vi "setUnderlineToDocument.vi"(8 "error in (no error)":errorcluster, 11 "xwpfRun in":refnum<class "xwpfRun.lvclass">) -> (0 "error out":errorcluster, 3 "xwpfRun out":refnum<class "xwpfRun.lvclass">)   [LabVIEW 2017, in "Word_Specific.lvlib" / "xwpfRun.lvclass"]
uses:
  xwpfRun.lvclass
  xwpfRun.lvclass/xwpfRun.ctl
  C:/Users/Neo/Desktop/Dev_Tools_BR/LabVIEW_NPOI/lib/NPOI 2.1.1/NPOI.OOXML.dll
  lib/NPOI 2.1.1/NPOI.OOXML.dll
  Styles/Style/Style.lvclass
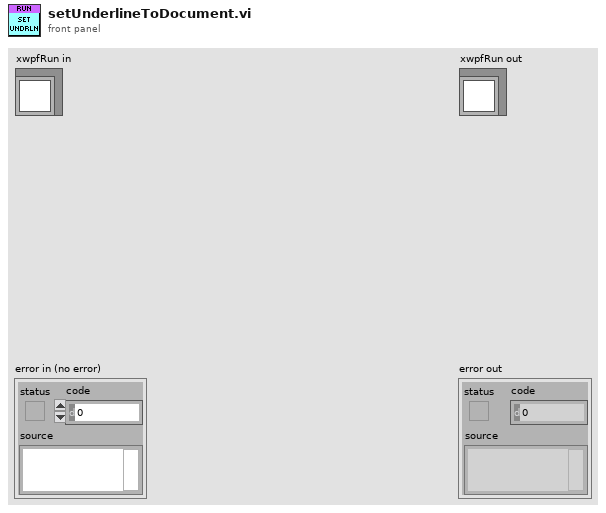
[diagram p1: front panel]
types:
  T1 = typedef "Styles.lvlib/Underline--ring.ctl" = i32
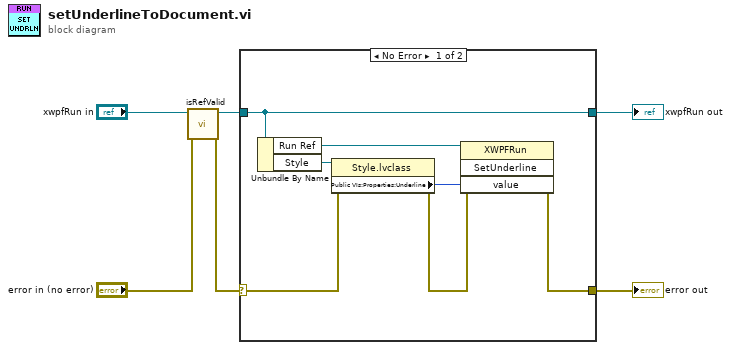
[diagram p0: block diagram]
diagram:
  n1 = call-dynamic "isRefValid.vi"("error in (no error)"="error in (no error)", "xwpfRun in"="xwpfRun in") -> ("error out"=w1:errorcluster, "xwpfRun out"=w3:refnum<class "xwpfRun.lvclass">)  [unwired: 8 in]
  n2 = case shown="No Error" w1 {
    selector: w1 -> [w12 w15]
    tunnel: [w10 w15] -> w6
    tunnel: [w9 w14] -> w4
    tunnel: w3 -> [w9 w14]
    frame No Error {
      n3 = Unbundle By Name(w9) -> ("Run Ref"=w7:refnum<k24>, "Style"=w13:refnum<class "Style.lvclass">)
      n4 = property class="Style.lvclass"(reference=w13, error in=w12) -> (error out=w11:errorcluster, "Public VIs:Properties:Underline"=w8:T1)  [unwired: 1 out]
      n5 = invoke class="XWPFRun" method="SetUnderline"(reference=w7, error in=w11, "value"=w8) -> (error out=w10:errorcluster)  [unwired: 1 in, 3 out]
    }
    frame Error {
    }
  }
  "error out" <- w6
  "xwpfRun out" <- w4
